vi "20kHzPWMDutyCycleGen.vi"(11 "output":i16) -> (3 "upper limit":i16)   [LabVIEW 2011]
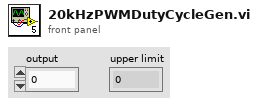
[diagram p1: front panel]
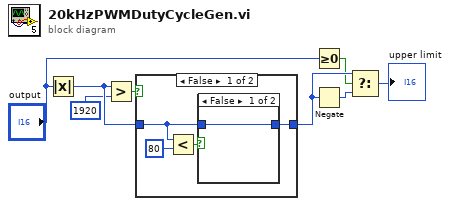
[diagram p0: block diagram]
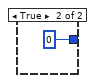
[diagram p2: hidden frame]
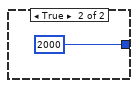
[diagram p3: hidden frame]
diagram:
  n1 = Absolute Value(x="output") -> (abs(x)=w6:i16)
  n2 = Greater?(x=w6, y=i16 1920) -> (0:w4:bool)
  n3 = case shown="False" w4 {
    tunnel: [w11 i16 2000] -> w5
    tunnel: w6 -> [w9 _]
    frame False {
      n4 = Less?(x=w9, y=i16 80) -> (x < y?=w10:bool)
      n5 = case shown="False" w10 {
        tunnel: [w13 i16 0] -> w11
        tunnel: w9 -> [w13 _]
        frame False {
        }
        frame True {
        }
      }
    }
    frame True {
    }
  }
  n6 = Greater Or Equal To 0?(x="output") -> (x >= 0?=w1:bool)
  n7 = Negate(x=w5) -> (-x=w2:i16)
  n8 = Select(t=w5, s=w1, f=w2) -> (s? t:f=→"upper limit":i16)
